vi "TFA Phase Vocoder Online (SubVI).vi"(8 "hop":i32=256, 9 "N":i32=256, 10 "squeeze":dbl=0.5, 11 "STFT coef in":cdb[][](array[numeric])=array513x15[7695 elements]) -> (3 "STFT coef out":cdb[][](array[numeric]))   [LabVIEW 2012]
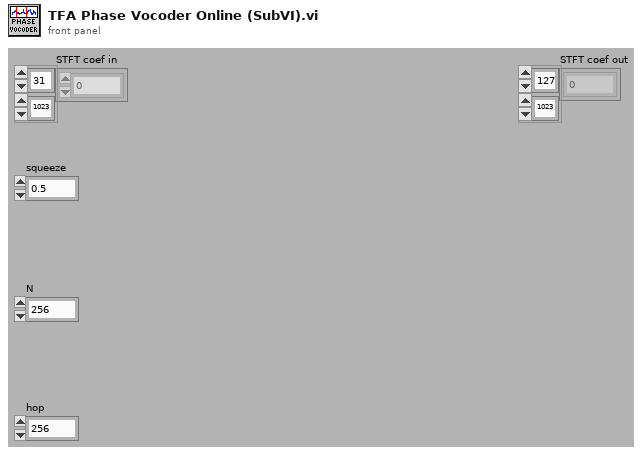
[diagram p1: front panel]
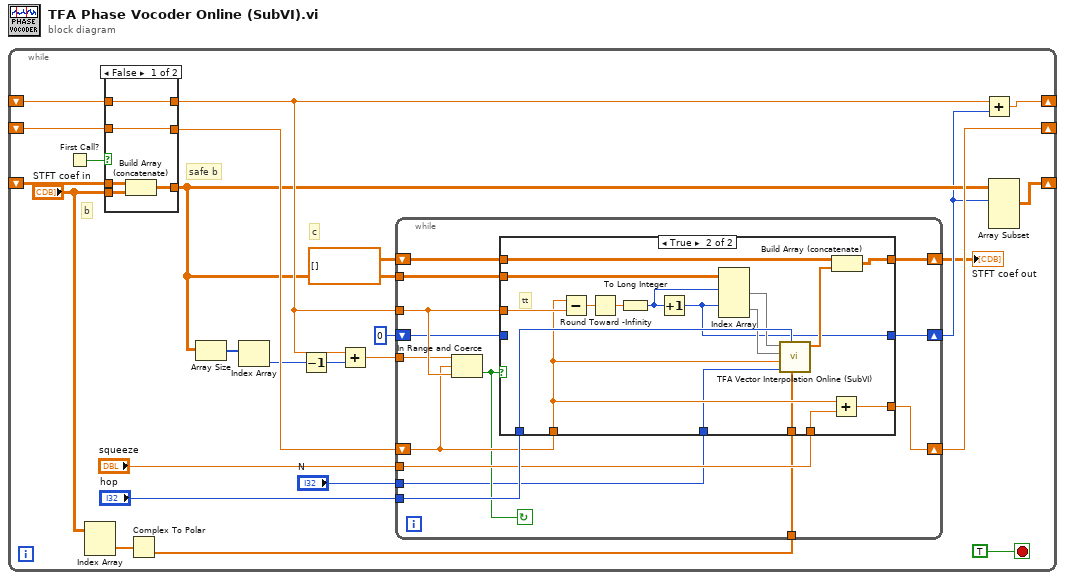
[diagram p0: block diagram]
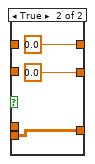
[diagram p3: hidden frame]
diagram:
  n1 = while {
    shift-right: [w19] -> _
    shift-left: _ -> [w20]
    shift-right: [w17] -> _
    shift-left: _ -> [w18]
    shift-right: [w8] -> _
    shift-left: _ -> [w16]
    stop <- TRUE stop-if-true
    # "c"
    # "b"
    # "safe b"
    n2 = First Call?() -> (First Call?: T/F=w22:bool)
    n3 = Index Array(array="STFT coef in") -> (element=w5:cdb[])  [unwired: 2 in]
    n4 = case shown="False" w22 {
      tunnel: [w64 0.0] -> w21
      tunnel: w20 -> [w64 _]
      tunnel: [w63 0.0] -> w14
      tunnel: w18 -> [w63 _]
      tunnel: "STFT coef in" -> [w61 w65]
      tunnel: [w60 w65] -> w9
      tunnel: w16 -> [w62 _]
      frame False {
        n5 = Build Array (concatenate)(w62, w61) -> (w60:cdb[][])
      }
      frame True {
      }
    }
    n6 = Complex To Polar(r * e^(i*theta)=w5) -> (theta=w4:dbl[])  [unwired: 1 out]
    n7 = Array Size(array=w9) -> (size(s)=w13:i32[])
    n8 = Index Array(array=w13) -> (element=w12:i32)  [unwired: 1 in]
    n9 = Decrement(x=w12) -> (x-1=w6:i32)
    n10 = Add(x=w14, y=w6) -> (x+y=w11:dbl)
    n11 = while {
      tunnel: "squeeze" -> [w30]
      shift-right: [w36] -> w2
      shift-left: cdb[][] [] ("initialized array") -> [w37]
      tunnel: "hop" -> [w39]
      shift-right: [w29] -> w19
      shift-left: w21 -> [w34]
      tunnel: w9 -> [w38]
      tunnel: w14 -> [w35]
      tunnel: w11 -> [w33]
      shift-right: [w32] -> w7
      shift-left: 0 -> [w31]
      tunnel: w4 -> [w27]
      tunnel: "N" -> [w26]
      stop <- w28 continue-if-true
      n12 = In Range and Coerce(upper limit=w33, x=w34, lower limit=w35) -> (In Range?=w28:bool)  [unwired: 1 out]
      n13 = case shown="True" w28 {
        tunnel: w39 -> [_ w59]
        tunnel: w38 -> [_ w56]
        tunnel: w37 -> [w41 w53]
        tunnel: [w41 w51] -> w36
        tunnel: w35 -> [_ w50]
        tunnel: w34 -> [w40 w47]
        tunnel: [w42 w48] -> w32
        tunnel: w31 -> [w42 _]
        tunnel: w30 -> [_ w46]
        tunnel: [w40 w45] -> w29
        tunnel: w27 -> [_ w44]
        tunnel: w26 -> [_ w43]
        frame False {
        }
        frame True {
          # "tt"
          n14 = Subtract(x=w47, y=w50) -> (x-y=w58:dbl)
          n15 = Round Toward -Infinity(1:w58) -> (0:w57:dbl)
          n16 = To Long Integer(number=w57) -> (32bit integer=w49:i32)
          n17 = Increment(x=w49) -> (x+1=w48:i32)
          n18 = Index Array(array=w56, index (row) #1=w49, index (row) #2=w48) -> (element #1=w55:cdb[], element #2=w54:cdb[])  [unwired: 2 in]
          n19 = call "TFA Vector Interpolation Online (SubVI).vi"("phase 0"=w44, "hop"=w59, "N"=w43, "new time instance (t)"=w47, "FFT (t1)"=w54, "FFT (t0)"=w55) -> ("interpolation"=w52:cdb[])  [unwired: 5 out]
          n20 = Add(x=w47, y=w46) -> (x+y=w45:dbl)
          n21 = Build Array (concatenate)(w53, w52) -> (w51:cdb[][])
        }
      }
    }
    "STFT coef out" <- w2
    n22 = Add(x=w14, y=w7) -> (x+y=w17:dbl)
    n23 = Array Subset(array=w9, index (row)=w7) -> (w8:cdb[][])  [unwired: 3 in]
  }
